vi "Create Log.vi"(8 "error in (no error)":errorcluster) -> (0 "error out":errorcluster, 3 "Log path":path)   [LabVIEW 2015]
uses:
  <vilib>/Utility/file.llb/Write Delimited Spreadsheet (string).vi
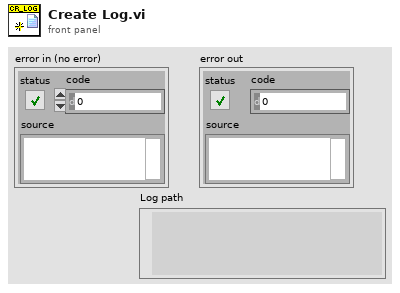
[diagram p1: front panel]
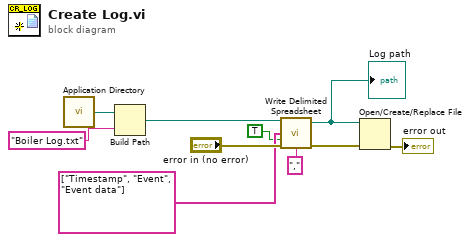
[diagram p0: block diagram]
diagram:
  n1 = call <vilib>:"Application Directory.vi"() -> ("Application Directory"=w1:path)
  n2 = Build Path(base path=w1, name or relative path="Boiler Log.txt") -> (appended path=w4:path)
  n3 = call-poly <vilib>:"Write Delimited Spreadsheet.vi"("file path (dialog if empty)"=w4, "1D data"=string[] ["Timestamp", "Event", "Event data"], "append to file? (F)"=TRUE, "error in (no error)"="error in (no error)", "delimiter (\\t)"="," ("delimiter (\\t)")) -> ("new file path (Not A Path if cancelled)"=w3:path, "error out"=w6:errorcluster)  [unwired: 9 in]
  "Log path" <- w3
  n4 = Open/Create/Replace File(file path (use dialog)=w3, error in=w6) -> (error out=→"error out":errorcluster)  [unwired: 4 in, 2 out]
